vi "Get Joystick.vi"(0 "refnum name":string="My Joystick RefNum") -> (2 "Axes":T2, 3 "Buttons":T1)   [LabVIEW 2014]
doc: "Converts code to use both the Logitech Extreme 3D Pro Joystick and the Logitech Attack 3 Joystick"
uses:
  <vilib>/Rock Robotics/WPI/Joystick/WPI_JoystickGetSetRefNum.vi
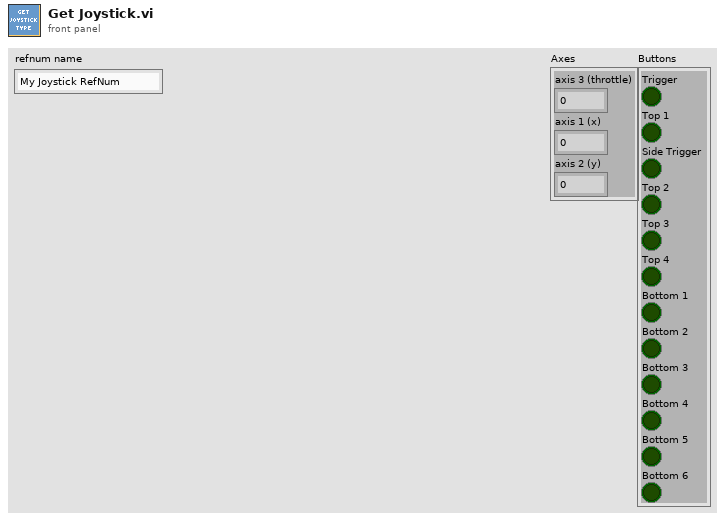
[diagram p1: front panel]
types:
  T1 = cluster{"Trigger":bool, "Top 1":bool, "Side Trigger":bool, "Top 2":bool, "Top 3":bool, "Top 4":bool, "Bottom 1":bool, "Bottom 2":bool, "Bottom 3":bool, "Bottom 4":bool, "Bottom 5":bool, "Bottom 6":bool}
  T2 = cluster{"axis 3 (throttle)":dbl, "axis 1 (x)":dbl, "axis 2 (y)":dbl}
  T3 = typedef "WPI_JoystickDevRef.ctl" = cluster{"Device":T4}
  T4 = typedef "WPI_JoystickDeviceEnum.ctl" = enum16{"USB 0", "USB 1", "USB 2", "USB 3", "USB 4", "USB 5"}
  T5 = cluster{"Button 1":bool, "Button 2":bool, "Button 3":bool, "Button 4":bool, "Button 5":bool, "Button 6":bool, "Button 7":bool, "Button 8":bool, "Button 9":bool, "Button 10":bool, "Button 11":bool, "Button 12":bool}
  T6 = cluster{"axis 1 (x)":dbl, "axis 2 (y)":dbl, "axis 3 (throttle)":dbl, "axis 4":dbl, "axis 5":dbl, "axis 6":dbl}
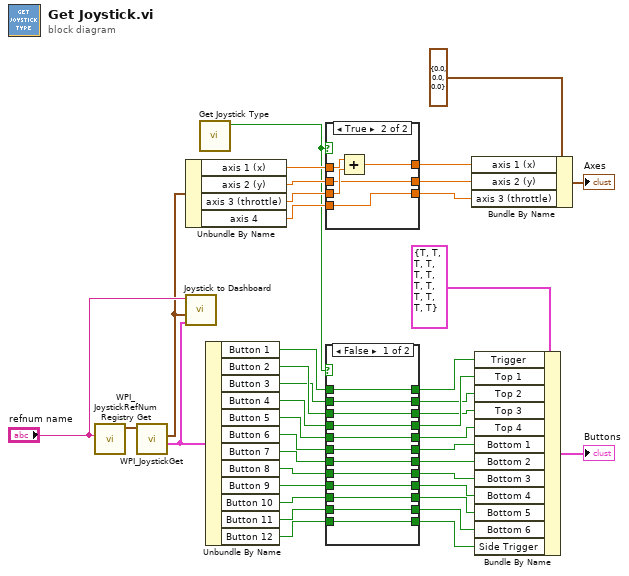
[diagram p0: block diagram]
diagram:
  n1 = call <vilib>:"WPI_JoystickRefNum Registry Get.vi"("refnum name"="refnum name") -> ("JoystickDevRef"=w40:T3)  [unwired: 9 in, 1 out]
  n2 = call <vilib>:"WPI_JoystickGet.vi"("JoystickDevRef"=w40) -> ("Buttons"=w2:T5, "Axes"=w3:T6)  [unwired: 4 in, 1 out]
  n3 = Unbundle By Name(w3) -> ("axis 1 (x)"=w39:dbl, "axis 2 (y)"=w38:dbl, "axis 3 (throttle)"=w37:dbl, "axis 4"=w36:dbl)
  n4 = call "Joystick to Dashboard.vi"("Raw Buttons"=w2, "Raw Axes"=w3, "refnum name"="refnum name") -> ()  [unwired: 9 in]
  n5 = call "Get Joystick Type.vi"() -> ("Joystick Type"=w1:bool)  [unwired: 11 in]
  n6 = Unbundle By Name(w2) -> ("Button 1"=w32:bool, "Button 2"=w30:bool, "Button 3"=w29:bool, "Button 4"=w28:bool, "Button 5"=w27:bool, "Button 6"=w26:bool, "Button 7"=w25:bool, "Button 8"=w24:bool, "Button 9"=w23:bool, "Button 10"=w22:bool, "Button 11"=w21:bool, "Button 12"=w20:bool)
  n7 = case shown="True" w1 {
    tunnel: w39 -> [w43 w48]
    tunnel: w38 -> [w42 w45]
    tunnel: w37 -> [w41 w47]
    tunnel: w36 -> [_ w44]
    tunnel: [w43 w46] -> w5
    tunnel: [w42 w45] -> w6
    tunnel: [w41 w44] -> w35
    frame False {
    }
    frame True {
      n8 = Add(x=w48, y=w47) -> (x+y=w46:dbl)
    }
  }
  n9 = case shown="False" w1 {
    tunnel: w32 -> [w60 w72]
    tunnel: [w60 w72] -> w31
    tunnel: w30 -> [w51 w71]
    tunnel: w29 -> [w50 w63]
    tunnel: w28 -> [w49 w62]
    tunnel: w27 -> [w52 w64]
    tunnel: w26 -> [w58 w61]
    tunnel: w25 -> [w57 w70]
    tunnel: w24 -> [w56 w69]
    tunnel: w23 -> [w55 w68]
    tunnel: w22 -> [w54 w67]
    tunnel: w21 -> [w53 w66]
    tunnel: w20 -> [w59 w65]
    tunnel: [w49 w64] -> w19
    tunnel: [w50 w63] -> w18
    tunnel: [w51 w62] -> w17
    tunnel: [w52 w61] -> w16
    tunnel: [w58 w70] -> w15
    tunnel: [w57 w69] -> w14
    tunnel: [w56 w68] -> w13
    tunnel: [w55 w67] -> w12
    tunnel: [w54 w66] -> w11
    tunnel: [w53 w65] -> w10
    tunnel: [w59 w71] -> w9
    frame False {
    }
    frame True {
    }
  }
  n10 = Bundle By Name(cluster=T2 {"axis 3 (throttle)"=0.0, "axis 1 (x)"=0.0, "axis 2 (y)"=0.0} ("input cluster"), "axis 1 (x)"=w5, "axis 2 (y)"=w6, "axis 3 (throttle)"=w35) -> (→"Axes":T2)
  n11 = Bundle By Name(cluster=T1 {"Trigger"=TRUE, "Top 1"=TRUE, "Side Trigger"=TRUE, "Top 2"=TRUE, "Top 3"=TRUE, "Top 4"=TRUE, "Bottom 1"=TRUE, "Bottom 2"=TRUE, "Bottom 3"=TRUE, "Bottom 4"=TRUE, "Bottom 5"=TRUE, "Bottom 6"=TRUE} ("input cluster"), "Trigger"=w31, "Top 1"=w19, "Top 2"=w18, "Top 3"=w17, "Top 4"=w16, "Bottom 1"=w15, "Bottom 2"=w14, "Bottom 3"=w13, "Bottom 4"=w12, "Bottom 5"=w11, "Bottom 6"=w10, "Side Trigger"=w9) -> (→"Buttons":T1)
